vi "Get Projects Section Enabled.vi"(8 "error in (no error)":errorcluster {"code" format="Error %.0f"}, 11 "VIDoc Parser In":refnum<class "VIDoc Parser.lvclass">) -> (0 "error out":errorcluster {"code" format="Error %.0f"}, 2 "Projects":bool=TRUE, 3 "VIDoc Parser Out":refnum<class "VIDoc Parser.lvclass">)   [LabVIEW 2023, in "VIDoc Parsing.lvlib" / "VIDoc Parser.lvclass"]
uses:
  VIDoc Parser.lvclass
  VIDoc Parser.lvclass/VIDoc Parser.ctl
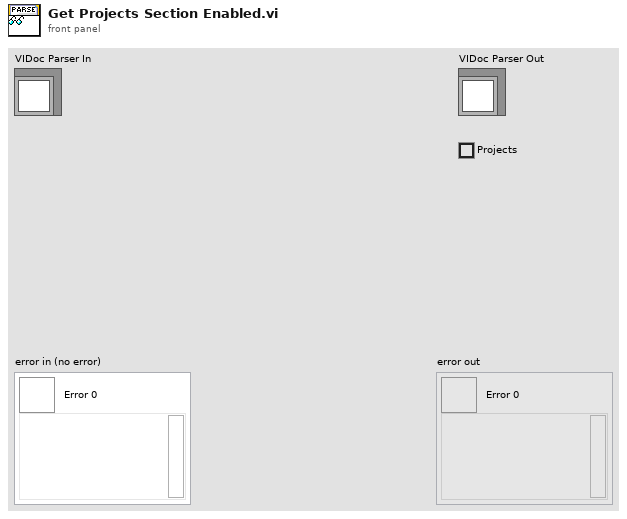
[diagram p1: front panel]
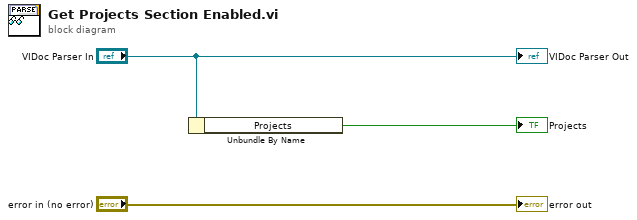
[diagram p0: block diagram]
diagram:
  n1 = Unbundle By Name("VIDoc Parser In") -> ("Projects"=→"Projects":bool)
  "error out" <- "error in (no error)"
  "VIDoc Parser Out" <- "VIDoc Parser In"
